vi "Run Tests (Path).vi"(7 "TextTestRunner in":refnum<class "TextTestRunner.lvclass">, 8 "error in (no error)":errorcluster, 10 "Test Path":path) -> (0 "error out":errorcluster, 1 "test details":string, 2 "successful?":bool)   [LabVIEW 2011, in "VI Tester API.lvlib"]
doc: "Run test classes (TestCase or TestSuites or LabVIEW project containing tests) by file path. Test Path is the file path to the *.lvclass or *.lvproj file on disk."
uses:
  VI Tester API.lvlib
  Classes/TextTestRunner/TextTestRunner.lvclass
  <userlib>/_OpenG.lib/file/file.llb/Strip Path Extension - Path__ogtk.vi
  Libraries/VITesterUtilities.lvlib
panel:
  # "JKI VI Tester for LabVIEW\nhttp://jkisoft.com/vi-tester\nCopyright (C) 2007-2009, JKI <info@jkisoft.com>\nALL RIGHTS RESERVED"
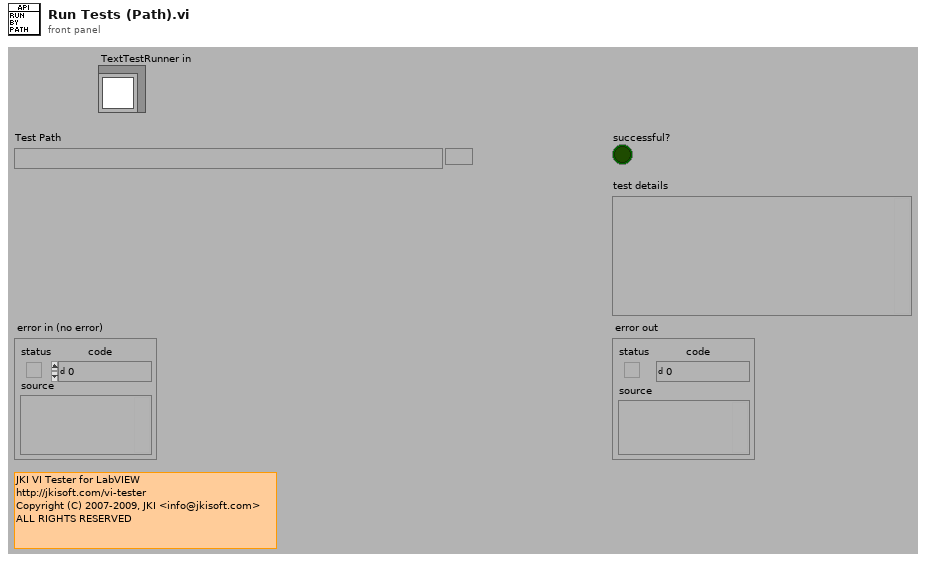
[diagram p1: front panel]
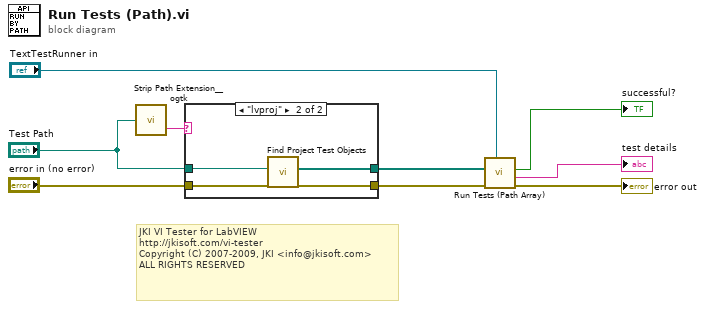
[diagram p0: block diagram]
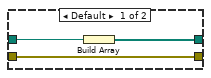
[diagram p2: hidden frame]
diagram:
  # "JKI VI Tester for LabVIEW\nhttp://jkisoft.com/vi-tester\nCopyright (C) 2007-2009, JKI <info@jkisoft.com>\nALL RIGHTS RESERVED"
  n1 = call-poly <userlib>:"Strip Path Extension__ogtk.vi"("path"="Test Path") -> ("extension"=w6:string)  [unwired: 1 out]
  n2 = case shown="\"lvproj\"" w6 {
    tunnel: [w11 w15] -> w4
    tunnel: "error in (no error)" -> [w11 w16]
    tunnel: "Test Path" -> [w12 w14]
    tunnel: [w10 w13] -> w2
    frame Default {
      n3 = Build Array(w12) -> (w10:path[])
    }
    frame "lvproj" {
      n4 = call "Find Project Test Objects.vi"("error in"=w16, "Project"=w14) -> ("error out"=w15:errorcluster, "TestPaths"=w13:path[])  [unwired: 8 in]
    }
  }
  n5 = call "Run Tests (Path Array).vi"("TextTestRunner in"="TextTestRunner in", "error in (no error)"=w4, "Test Paths"=w2) -> ("error out"=→"error out":errorcluster, "test details"=→"test details":string, "successful?"=→"successful?":bool)  [unwired: 6 in]
